vi "display_data.vi"() -> ()   [LabVIEW 2013]
uses:
  <vilib>/Analysis/NI_AALBase.lvlib
panel:
  out "Histogram":dynamicdata(graph)
  out "Histogram 3":dynamicdata(graph) caption="Histogram"
  in  "First File to read":path
  out "Numeric":i32
  out "path":path
  out "List of All the File Names":string[](array[string])
  out "Waveform Graph 2":dbl[](graph)
  out "median 2":dbl format="%0.2f"
  out "Waveform Graph":dbl[](graph)
  in  "data points":i32
  in  "seconds to wait":u32
  out "XY Graph 2":cluster{sgl[], sgl[]}(graph)
  in  "par2 2":i32
  in  "par1 2":i32
  out "XY GRAPH":cluster{sgl[], sgl[]}(graph)
  in  "par2":i32
  in  "par1":i32
  out "median":dbl format="%0.2f"
  in  "Diva Directory":path=path "C:/Program Files/National Instruments/LabVIEW 7.0"
  in  "error in":errorcluster
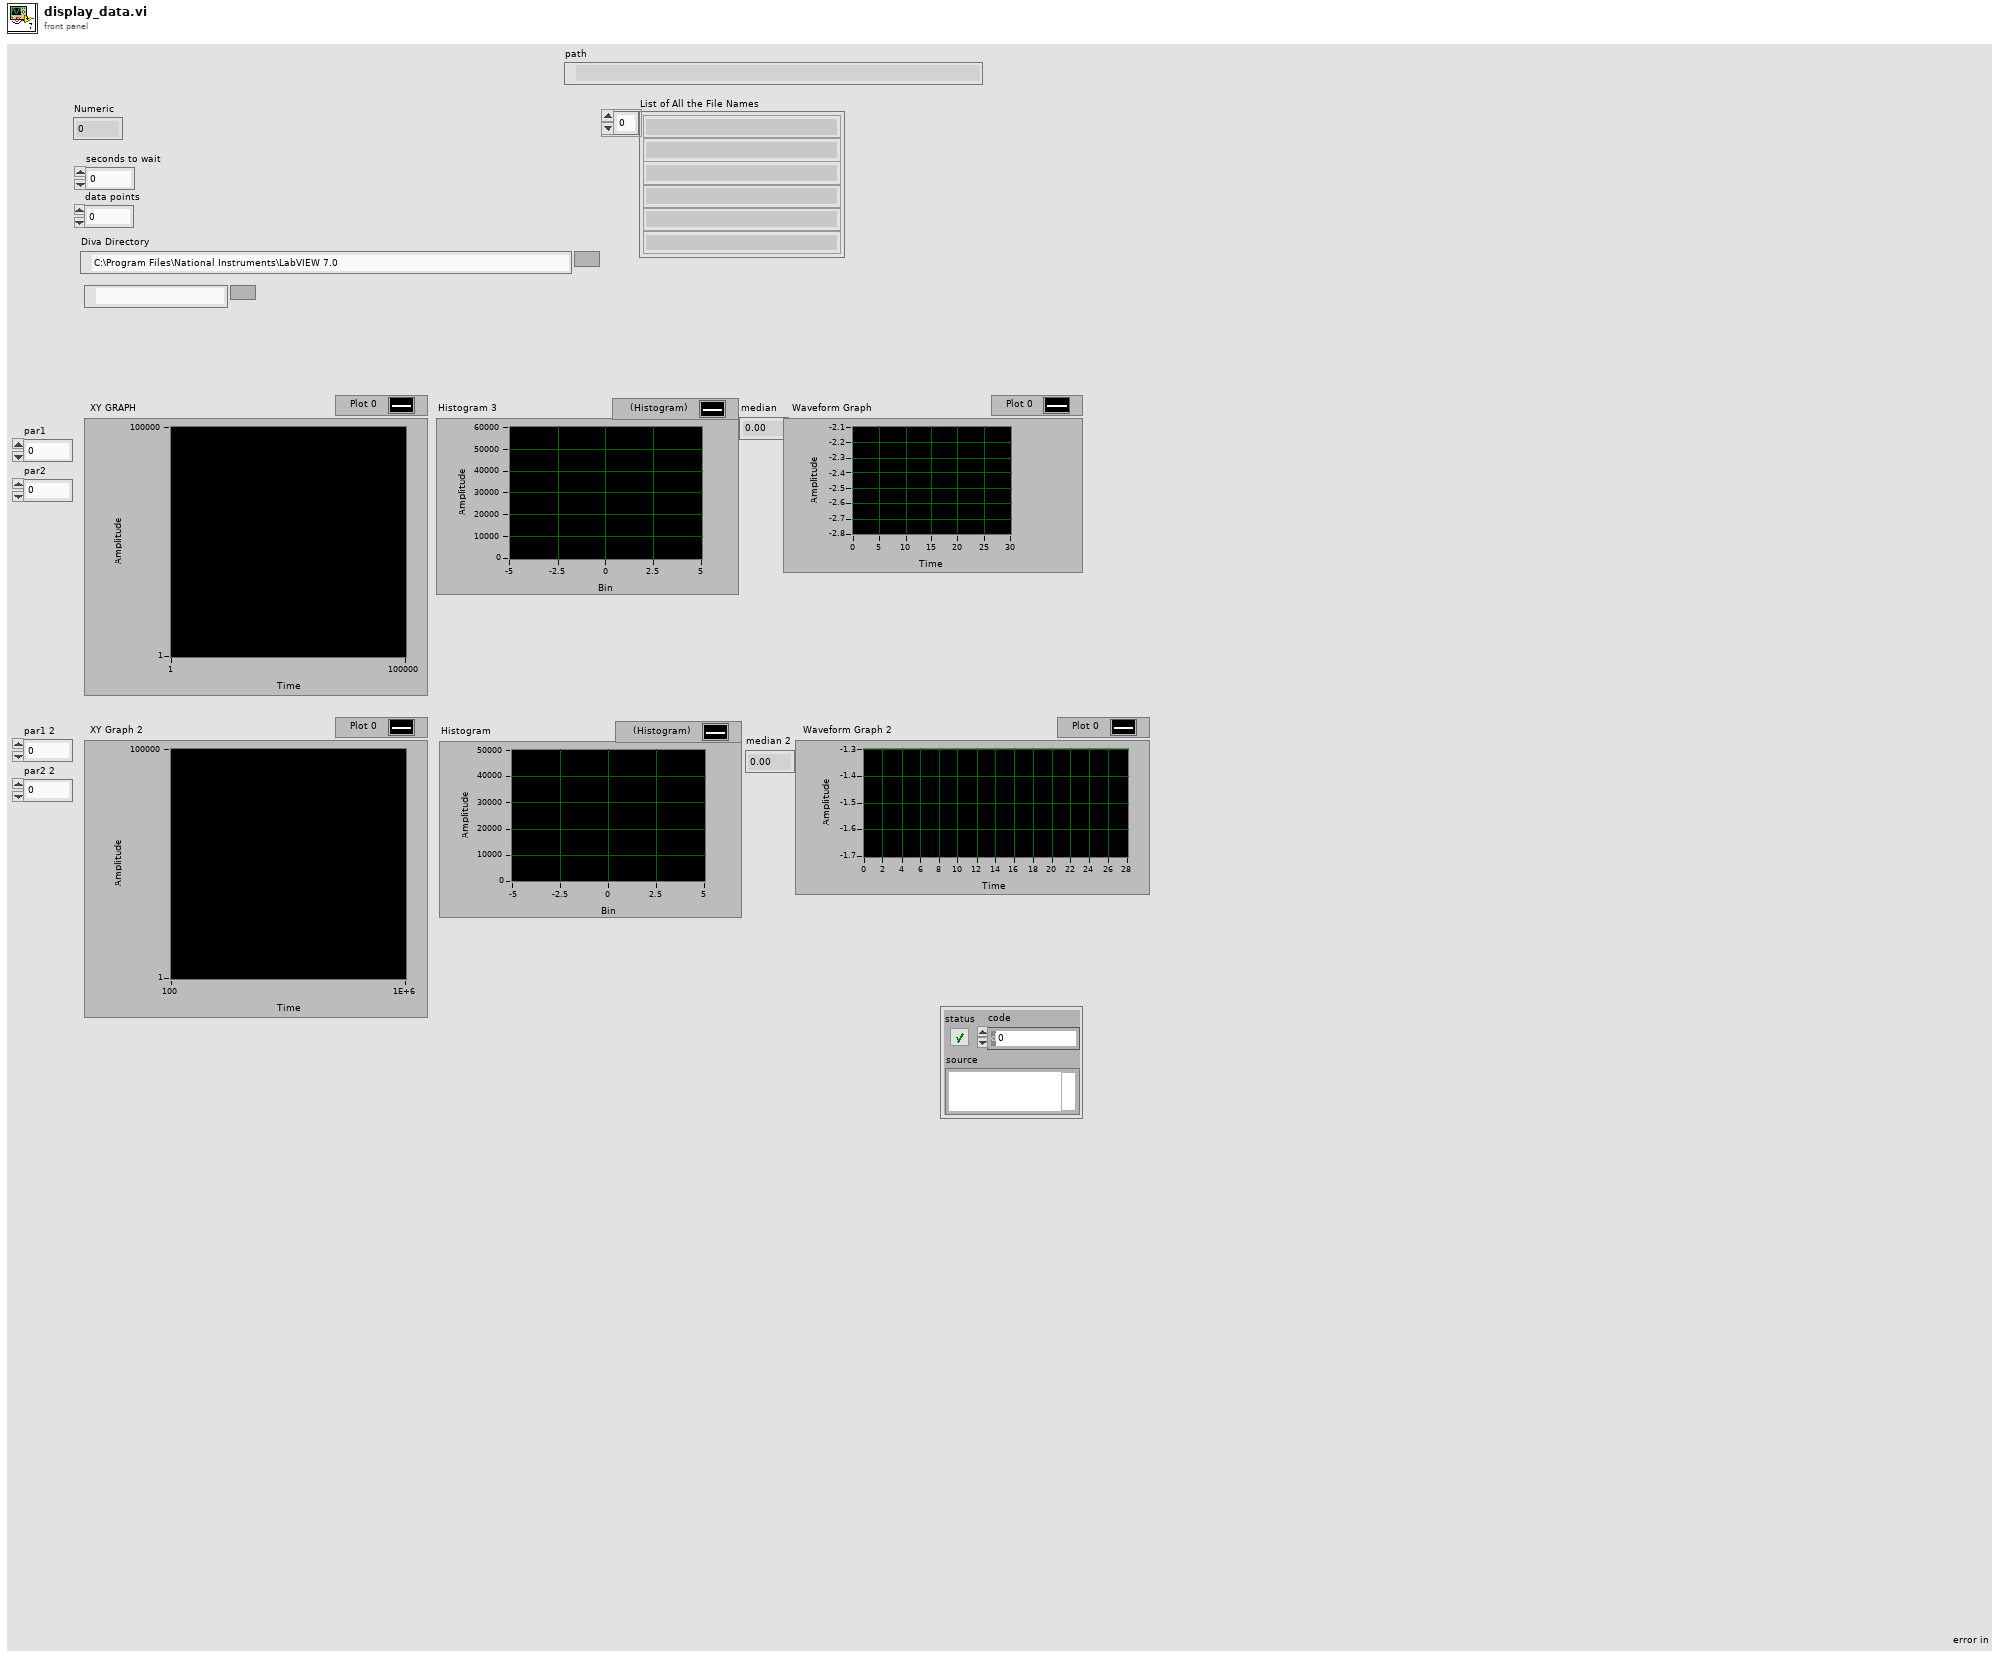
[diagram p1: front panel]
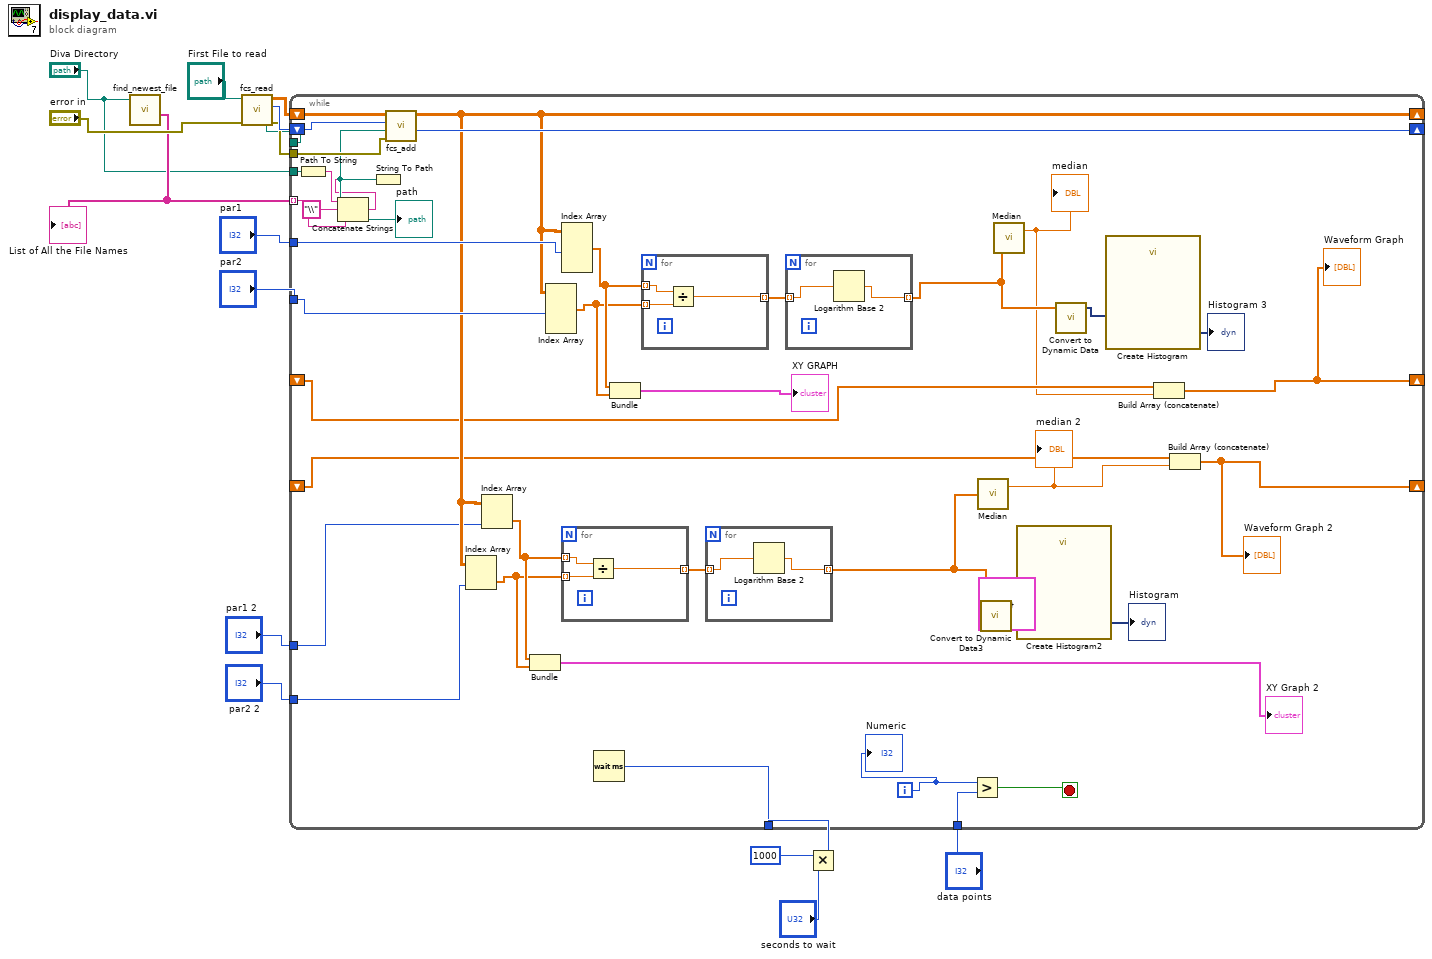
[diagram p0: block diagram]
diagram:
  n1 = call "find_newest_file.vi"("Directory Path to Start the Search"="Diva Directory") -> ("List of All the File Names"=w3:string[])  [unwired: 7 in, 2 out]
  "List of All the File Names" <- w3
  n2 = call "fcs_read.vi"("error in (no error)"="error in", "Path"="First File to read") -> ("error out"=w12:errorcluster, "byte offset"=w14:i64, "Array"=w13:sgl[][])  [unwired: 6 in, 1 out]
  n3 = Multiply(x=u32 1000, y="seconds to wait") -> (x*y=w5:u32)
  n4 = while {
    tunnel: "First File to read" -> [_]
    shift-right: [w42] -> _
    shift-left: w13 -> [w54]
    shift-right: [w51] -> _
    shift-left: w14 -> [w53]
    tunnel: w12 -> [w52]
    tunnel: "par1" -> [w49]
    tunnel: "par2" -> [w48]
    tunnel: "par1 2" -> [w41]
    tunnel: "par2 2" -> [w40]
    tunnel: w5 -> [w39]
    tunnel: "data points" -> [w38]
    tunnel: w3 -> [w33] mode=indexing
    tunnel: "Diva Directory" -> [w35]
    shift-right: [w20] -> _
    shift-left: _ -> [w22]
    shift-right: [w16] -> _
    shift-left: _ -> [w19]
    i -> [w23]
    stop <- w37 stop-if-true
    (unwired) cluster{sgl[], sgl[]} {[], []} ("WAITING PLOT")
    n5 = Path To String(path=w35) -> (string=w34:string)
    n6 = Concatenate Strings(w34, "\\" ("string"), w33) -> (w31:string)
    n7 = String To Path(string=w31) -> (path=w36:path)
    "path" <- w36
    n8 = call "fcs_add.vi"("Array in"=w54, "byte offset in"=w53, "Path in"=w36, "error in (no error)"=w52) -> ("total data"=w42:sgl[][], "byte offset out"=w51:i64)  [unwired: 2 in, 2 out]
    n9 = Index Array(array=w42, index (col)=w40) -> (element=w43:sgl[])  [unwired: 1 in]
    n10 = Index Array(array=w42, index (col)=w41) -> (element=w44:sgl[])  [unwired: 1 in]
    n11 = Bundle("total data"=w44, "total data"=w43) -> (→"XY Graph 2":cluster{"total data":sgl[], "total data":sgl[]})  [unwired: 1 in]
    n12 = Index Array(array=w42, index (col) #1=w48) -> (element #1=w46:sgl[])  [unwired: 3 in, 1 out]
    n13 = Index Array(array=w42, index (col) #1=w49) -> (element #1=w47:sgl[])  [unwired: 3 in, 1 out]
    n14 = for {
      tunnel: w43 -> [w59] mode=indexing
      tunnel: [w57] -> w45 mode=indexing
      tunnel: w44 -> [w58] mode=indexing
      n15 = Divide(x=w58, y=w59) -> (x/y=w57:sgl)
    }
    n16 = Wait (ms)(milliseconds to wait=w39) -> ()  [unwired: 1 out]
    n17 = Bundle("total data"=w47, "total data"=w46) -> (→"XY GRAPH":cluster{"total data":sgl[], "total data":sgl[]})  [unwired: 1 in]
    n18 = for {
      tunnel: w46 -> [w64] mode=indexing
      tunnel: [w62] -> w50 mode=indexing
      tunnel: w47 -> [w63] mode=indexing
      n19 = Divide(x=w63, y=w64) -> (x/y=w62:sgl)
    }
    n20 = for {
      tunnel: w45 -> [w56] mode=indexing
      tunnel: [w55] -> w26 mode=indexing
      n21 = Logarithm Base 2(1:w56) -> (0:w55:sgl)
    }
    n22 = for {
      tunnel: w50 -> [w61] mode=indexing
      tunnel: [w60] -> w30 mode=indexing
      n23 = Logarithm Base 2(1:w61) -> (0:w60:sgl)
    }
    n24 = Greater?(x=w23, y=w38) -> (0:w37:bool)
    n25 = call <vilib>:"Median.vi"("X"=w26) -> ("median"=w21:dbl)  [unwired: 1 out]
    "median 2" <- w21
    n26 = call "Convert to Dynamic Data3"("Array"=w26) -> ("Dynamic Data Type"=w25:dynamicdata)  [unwired: 3 in]
    n27 = call <vilib>:"Median.vi"("X"=w30) -> ("median"=w18:dbl)  [unwired: 1 out]
    "median" <- w18
    n28 = call "Create Histogram2"("Signal"=w25) -> ("Histogram"=→"Histogram":dynamicdata)  [unwired: 9 in, 1 out]
    n29 = call "Convert to Dynamic Data"("Array"=w30) -> ("Dynamic Data Type"=w29:dynamicdata)  [unwired: 3 in]
    n30 = call "Create Histogram"("Signal"=w29) -> ("Histogram"=→"Histogram 3":dynamicdata)  [unwired: 9 in, 1 out]
    n31 = Build Array (concatenate)(w19, w18) -> (w16:dbl[])
    "Waveform Graph" <- w16
    n32 = Build Array (concatenate)(w22, w21) -> (w20:dbl[])
    "Waveform Graph 2" <- w20
    "Numeric" <- w23
  }
